vi "OCV Target Server.vi"   [LabVIEW 2019]
uses:
  <vilib>/NI/STM/SubVIs/MetaDataElement.ctl
  <vilib>/NI/STM/TCP/Write Meta Data (TCP Ref).vi
  <vilib>/NI/STM/TCP/Get Connection Reference (TCP).vi
  <vilib>/NI/STM/TCP/Write Meta Data (TCP Clst).vi
  <vilib>/NI/STM/TCP/Write Message (TCP).vi
  <vilib>/NI/STM/TCP/Read Message (TCP).vi
  <vilib>/NI/STM/NI STM.lvlib
types:
  T1 = typedef "NI STM.lvlib/MetaDataElement.ctl" = string
  T2 = typedef "NI STM.lvlib/TCP Connection Info.ctl" = cluster{"connection ID":refnum<k5>, "meta data":T1[]}
  T3 = cluster{"V ch0 Array":dbl[], "V ch1 Array":dbl[], "V ch2 Array":dbl[], "V ch3 Array":dbl[], "V ch4 Array":dbl[], "Elapsed Time (ms)":u32, "DMM Fault Array":bool[]}
  T4 = typedef "OCVResults.ctl" = cluster{"V ch0 Array":dbl[], "V ch1 Array":dbl[], "V ch2 Array":dbl[], "V ch3 Array":dbl[], "V ch4 Array":dbl[], "Elapsed Time (ms)":u32, "DMM Fault Array":bool[]}
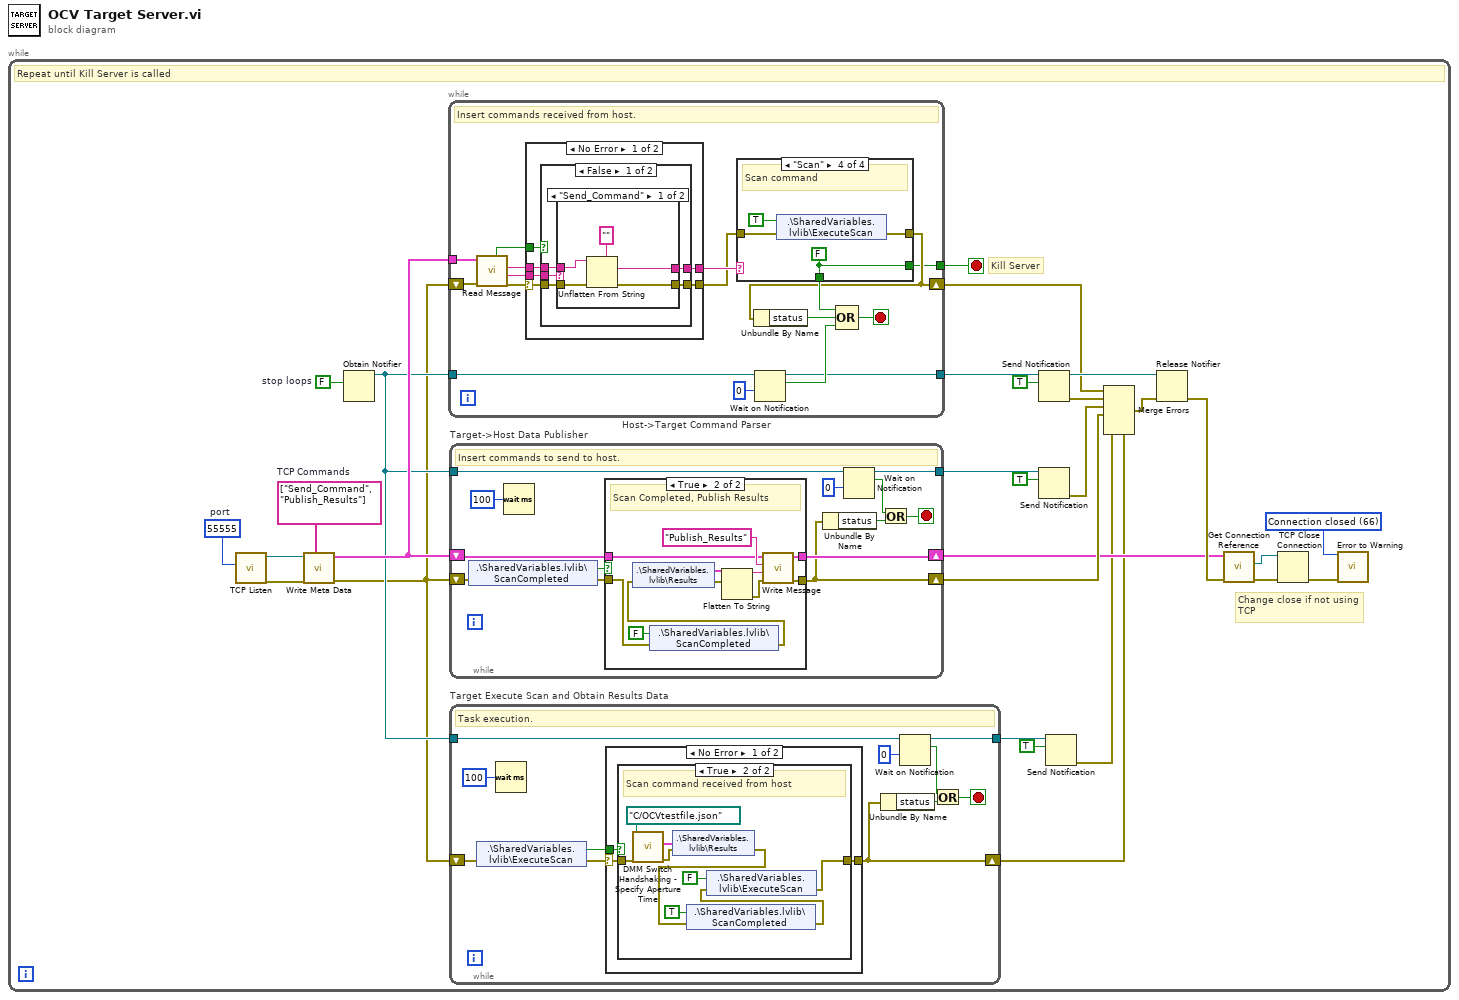
[diagram p0: block diagram]
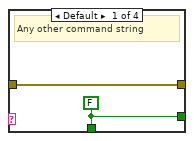
[diagram p5: hidden frame]
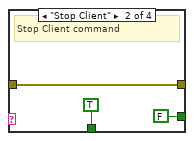
[diagram p6: hidden frame]
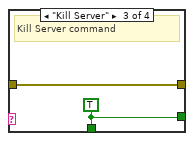
[diagram p7: hidden frame]
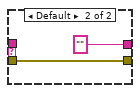
[diagram p8: hidden frame]
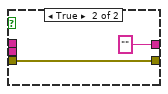
[diagram p9: hidden frame]
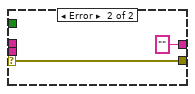
[diagram p10: hidden frame]
diagram:
  n1 = while {
    stop <- w1 stop-if-true
    w17 = FALSE  # stop loops
    w11 = T1[] ["Send_Command", "Publish_Results"]  # TCP Commands
    w28 = 66 items=["No Error", "Argument Error", "Memory Full", "Out of Zone", "End of File", "File Already Open", "Generic File IO Error", "File Not Found", "File Permission Error", "Disk Full", "Duplicate Path", "Too Many Files Open", "Not Enabled", "Resource File Not Found", "Cannot Add Resource", "Resource Not Found", "Image Not Found", "Image Memory Error", "Pen Does Not Exist", "Config Bad Type", "Config Token Not Found", "Config Parse Error", "Config Memory Error", "Bad External Code Format", "Bad External Code Offset", "External Code Not Present", "Null Window", "Destroy Window Mixup", "Null Menu", "Print Aborted", "Bad Print Record", "Print Driver Error", "Windows Error During Print", "Memory Error During Print", "Print Dialog Error", "Generic Print Error", "Invalid Device Refnum", "Device Not Found", "Device Parameter Error", "Device Unit Error", "Can't Open Device", "Device Call Aborted", "Generic Error", "Cancelled By User", "Object ID Too Low", "Object ID Too High", "Object Not In Heap", "Unknown Heap", "Bad DefProc ID", "DefProc Not In Table", "Message Out Of Range", "Null Method", "Unknown Message", "Manager Call Not Supported", "Bad address", "Connection In progress", "Connection timed out", "Connection is already in progress", "Network attribute not supported", "Network error", "Address in use", "System out of memory", "Connection aborted", "Connection refused", "Connection is not connected", "Connection is already connected", "Connection closed", "Initialize error (interapplication manager)", "Bad occurrence", "Wait on unbound occurrence handler", "Occurrence queue overflow", "Bad path", "Semaphore not signaled", "Unrecognized type (interapplication manager)"] ("1st Error to Convert")
    w8 = u16 55555  # port
    # "Kill Server"
    # "Change close if not using TCP"
    # "Repeat until Kill Server is called"
    n2 = call <vilib>:"TCP Listen.vi"("port"=w8) -> ("error out"=w9:errorcluster, "connection ID"=w16:refnum<k5>)  [unwired: 3 in, 6 out]
    n3 = call-poly <vilib>:"Write Meta Data.vi"("meta data"=w11, "error in"=w9, "connection ID"=w16) -> ("error out"=w3:errorcluster, "connection info out"=w10:T2)  [unwired: 2 in, 5 out]
    n4 = Obtain Notifier(notification data type=w17) -> (notifier out=w7:refnum<notifier>)  [unwired: 3 in, 2 out]
    n5 = while "Host->Target Command Parser" {
      tunnel: w10 -> [w97]
      shift-right: [w82] -> w15
      shift-left: w3 -> [w96]
      tunnel: w7 -> [w90]
      tunnel: [w87] -> w19
      tunnel: [w81] -> w1
      stop <- w86 stop-if-true
      # "Insert commands received from host."
      n6 = call-poly <vilib>:"Read Message.vi"("error in"=w96, "connection info in"=w97) -> ("error out"=w92:errorcluster, "name"=w95:T1, "data string"=w94:string, "timed out?"=w93:bool)  [unwired: 3 in, 3 out]
      n7 = case shown="No Error" w92 {
        selector: w92 -> [w111 w130]
        tunnel: w95 -> [w114 _]
        tunnel: w94 -> [w113 _]
        tunnel: w93 -> [w112 _]
        tunnel: [w110 w130] -> w83
        tunnel: [w109 "" ("Message")] -> w85
        frame No Error {
          n8 = case shown="False" w112 {
            tunnel: w114 -> [w116 _]
            tunnel: w113 -> [w119 _]
            tunnel: w111 -> [w118 w128]
            tunnel: [w117 w128] -> w110
            tunnel: [w115 "" ("Message")] -> w109
            frame False {
              n9 = case shown="\"Send_Command\"" w116 {
                tunnel: w119 -> [w124 _]
                tunnel: w118 -> [w123 w126]
                tunnel: [w121 w126] -> w117
                tunnel: [w122 "" ("Message")] -> w115
                frame "Send_Command" {
                  n10 = Unflatten From String(type="" ("Message"), binary string=w124, error in (no error)=w123) -> (value=w122:string, error out=w121:errorcluster)  [unwired: 1 in, 2 out]
                }
                frame Default {
                }
              }
            }
            frame True {
            }
          }
        }
        frame Error {
        }
      }
      n11 = case shown="\"Scan\"" w85 {
        tunnel: [w98 TRUE ("value") w103 w105] -> w84
        tunnel: w83 -> [w99 w101 w104 w107]
        tunnel: [w99 w101 w104 w106] -> w82
        tunnel: [w98 FALSE ("value") w103 w105] -> w81
        frame Default {
          w98 = FALSE ("value")
          # "Any other command string"
        }
        frame "Stop Client" {
          # "Stop Client command"
        }
        frame "Kill Server" {
          w103 = TRUE ("value")
          # "Kill Server command"
        }
        frame "Scan" {
          w105 = FALSE ("value")
          # "Scan command"
          n12 = shared-variable ".\\SharedVariables.lvlib\\ExecuteScan"(TRUE ("Execute Scan"), error in=w107) -> (error out=w106:errorcluster)
        }
      }
      n13 = Unbundle By Name(w82) -> ("status"=w89:bool)
      n14 = Wait on Notification(notifier=w90, timeout in ms (-1)=0) -> (notifier out=w87:refnum<notifier>, notification=w88:bool)  [unwired: 2 in, 2 out]
      n15 = Compound Arithmetic op=OR(w84, w89, w88) -> (w86:bool)
    }
    n16 = while "Target->Host Data Publisher" {
      shift-right: [w58] -> w24
      shift-left: w3 -> [w55]
      shift-right: [w60] -> w12
      shift-left: w10 -> [w59]
      tunnel: w7 -> [w66]
      tunnel: [w62] -> w21
      stop <- w63 stop-if-true
      # "Insert commands to send to host."
      n17 = shared-variable ".\\SharedVariables.lvlib\\ScanCompleted"(error in=w55) -> (w57:bool, error out=w56:errorcluster)
      n18 = Wait (ms)(milliseconds to wait=u32 100) -> ()  [unwired: 1 out]
      n19 = case shown="True" w57 {
        tunnel: [w69 w78] -> w60
        tunnel: w59 -> [w69 w77]
        tunnel: w56 -> [w68 w73]
        tunnel: [w68 w76] -> w58
        frame False {
          # "Scan not completed"
        }
        frame True {
          # "Scan Completed, Publish Results"
          n20 = shared-variable ".\\SharedVariables.lvlib\\ScanCompleted"(FALSE ("Scan Completed?"), error in=w73) -> (error out=w70:errorcluster)
          n21 = shared-variable ".\\SharedVariables.lvlib\\Results"(error in=w70) -> (w72:T3, error out=w71:errorcluster)
          n22 = Flatten To String(anything=w72, error in (no error)=w71) -> (data string=w79:string, error out=w75:errorcluster)  [unwired: 1 in, 2 out]
          n23 = call-poly <vilib>:"Write Message.vi"("error in"=w75, "data"=w79, "name"="Publish_Results" ("Name"), "connection info in"=w77) -> ("error out"=w76:errorcluster, "connection info out"=w78:T2)  [unwired: 1 in, 5 out]
        }
      }
      n24 = Unbundle By Name(w58) -> ("status"=w64:bool)
      n25 = Wait on Notification(notifier=w66, timeout in ms (-1)=0) -> (notifier out=w62:refnum<notifier>, notification=w65:bool)  [unwired: 2 in, 2 out]
      n26 = Or(x=w65, y=w64) -> (x .or. y?=w63:bool)
    }
    n27 = while "Target Execute Scan and Obtain Results Data" {
      shift-right: [w33] -> w2
      shift-left: w3 -> [w30]
      tunnel: w7 -> [w39]
      tunnel: [w35] -> w5
      stop <- w36 stop-if-true
      # "Task execution."
      n28 = shared-variable ".\\SharedVariables.lvlib\\ExecuteScan"(error in=w30) -> (w32:bool, error out=w31:errorcluster)
      n29 = Wait (ms)(milliseconds to wait=u32 100) -> ()  [unwired: 1 out]
      n30 = case shown="No Error" w31 {
        selector: w31 -> [w42 w54]
        tunnel: [w41 w54] -> w33
        tunnel: w32 -> [w43 _]
        frame No Error {
          n31 = case shown="True" w43 {
            tunnel: w42 -> [w44 w53]
            tunnel: [w44 w51] -> w41
            frame False {
              # "Scan command not received from host"
            }
            frame True {
              # "Scan command received from host"
              n32 = call "DMM Switch Handshaking - Specify Aperture Time.vi"("error in"=w53, "file path (use dialog)"=path "C:/OCVtestfile.json") -> ("error out"=w45:errorcluster, "Results"=w47:T4)  [unwired: 8 in]
              n33 = shared-variable ".\\SharedVariables.lvlib\\Results"(w47, error in=w45) -> (error out=w46:errorcluster)
              n34 = shared-variable ".\\SharedVariables.lvlib\\ScanCompleted"(TRUE ("Execute Scan"), error in=w46) -> (error out=w48:errorcluster)
              n35 = shared-variable ".\\SharedVariables.lvlib\\ExecuteScan"(FALSE ("Execute Scan"), error in=w48) -> (error out=w51:errorcluster)
            }
          }
        }
        frame Error {
        }
      }
      n36 = Unbundle By Name(w33) -> ("status"=w37:bool)
      n37 = Wait on Notification(notifier=w39, timeout in ms (-1)=0) -> (notifier out=w35:refnum<notifier>, notification=w38:bool)  [unwired: 2 in, 2 out]
      n38 = Or(x=w38, y=w37) -> (x .or. y?=w36:bool)
    }
    n39 = Send Notification(notification=TRUE, notifier=w19) -> (notifier out=w25:refnum<notifier>, error out=w22:errorcluster)  [unwired: 1 in]
    n40 = Send Notification(notification=TRUE, notifier=w21) -> (error out=w23:errorcluster)  [unwired: 1 in, 1 out]
    n41 = Send Notification(notification=TRUE, notifier=w5) -> (error out=w4:errorcluster)  [unwired: 1 in, 1 out]
    n42 = Merge Errors(w15, w22, w23, w24, w4, w2) -> (w26:errorcluster)
    n43 = Release Notifier(notifier=w25, error in (no error)=w26) -> (error out=w27:errorcluster)  [unwired: 1 in, 2 out]
    n44 = call-poly <vilib>:"Get Connection Reference.vi"("error in"=w27, "connection info in"=w12) -> ("error out"=w14:errorcluster, "connection ID out"=w13:refnum<k5>)  [unwired: 8 out]
    n45 = TCP Close Connection(connection ID=w13, error in (no error)=w14) -> (error out=w29:errorcluster)  [unwired: 2 out]
    n46 = call <vilib>:"Error to Warning.vi"("1st Error to Convert"=w28, "error in"=w29) -> ()  [unwired: 3 in, 11 out]
  }
